vi "Dialog.vi"() -> (3 "Cancelled?":bool)   [LabVIEW 2013, in "TestVIs.lvlib"]
doc: "Use this template to create a dialog box with event handling."
uses:
  TestVIs.lvlib
panel:
  in  "Cancel":bool
  in  "OK":bool
  # "Add the contents of your dialog here.\n\nTip: use controls from the System category of the Controls \npalette for professional appearance.\n\nReplace this text with your own, or delete this label."
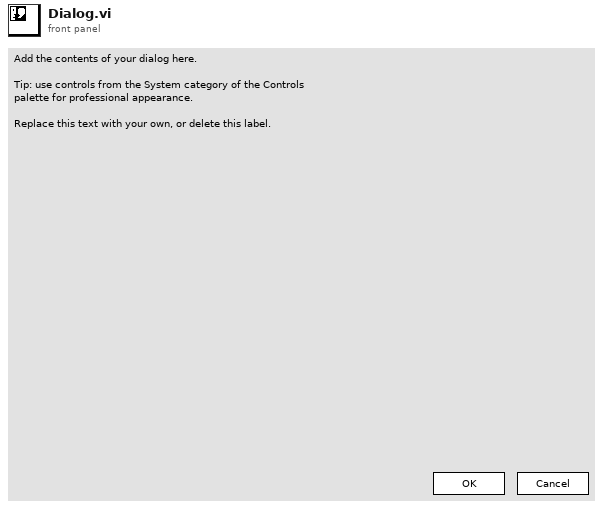
[diagram p1: front panel]
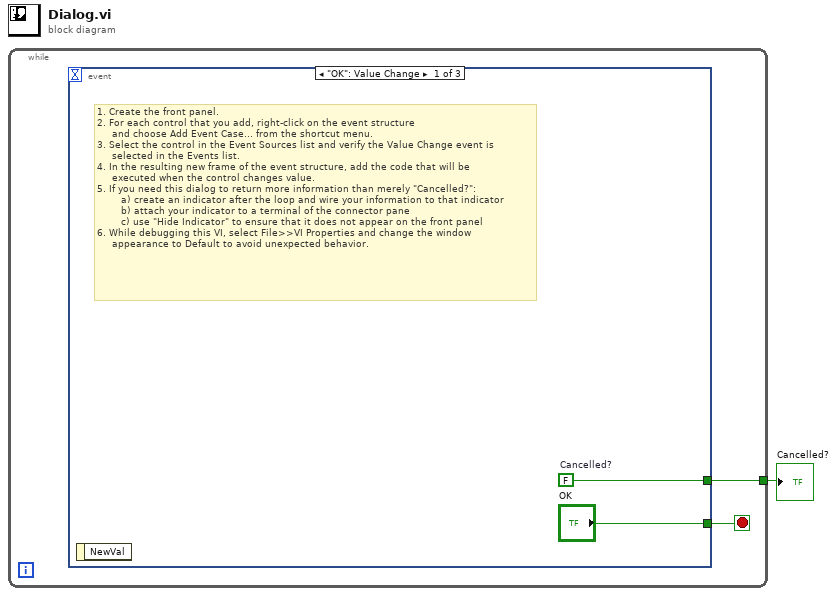
[diagram p0: block diagram]
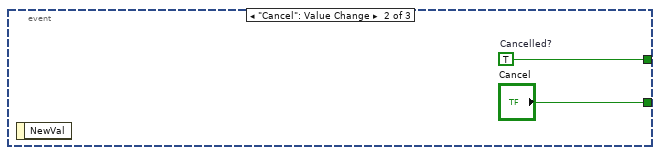
[diagram p2: hidden frame]
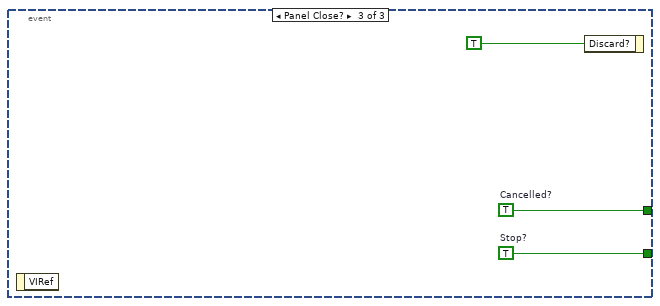
[diagram p3: hidden frame]
diagram:
  n1 = while {
    tunnel: [w2] -> w1
    stop <- w3 stop-if-true
    n2 = event shown="[0] \"OK\": Value Change" {
      selector: _ -> [_ _ _]
      dyn-events: _ -> [_ _ _]
      timeout: _ -> [_ _ _]
      tunnel: ["OK" "Cancel" w9] -> w3
      tunnel: [w5 w7 w8] -> w2
      event "OK": Value Change {
        w5 = FALSE  # Cancelled?
        # "1. Create the front panel.\n2. For each control that you add, right-click on the event structure \n     and choose Add Event Case... from the shortcut menu.\n3. Select the control in the Event Sources list and verify the Value Change event is \n     selected in the Events list.\n4. In the resulting new frame of the event structure, add the code that will be \n     executed when the control changes value.\n5. If you need this dialog to return more information than merely \"Cancelled?\":\n        a) create an indicator after the loop and wire your information to that indicator\n        b) attach your indicator to a terminal of the connector pane\n        c) use \"Hide Indicator\" to ensure that it does not appear on the front panel\n6. While debugging this VI, select File>>VI Properties and change the window \n     appearance to Default to avoid unexpected behavior."
        n3 = event-data() -> ()  [unwired: 1 in, 1 out]
      }
      event "Cancel": Value Change {
        w7 = TRUE  # Cancelled?
        n4 = event-data() -> ()  [unwired: 1 in, 1 out]
      }
      event Panel Close? {
        w8 = TRUE  # Cancelled?
        w9 = TRUE  # Stop?
        n5 = event-data() -> ()  [unwired: 1 in, 1 out]
        n6 = event-data("Discard?"=TRUE) -> ()  [unwired: 1 in, 1 out]
      }
    }
  }
  "Cancelled?" <- w1
